vi "Init.vi"(8 "error in (no error)":errorcluster, 11 "Laser View in":refnum<class "Laser View.lvclass">) -> (0 "error out":errorcluster, 3 "Laser View out":refnum<class "Laser View.lvclass">)   [LabVIEW 2022 SP3, in "Laser View.lvclass"]
uses:
  Laser View.lvclass
  Data.ctl
  Laser View.lvclass/Laser View.ctl
  iView/base view/base view.lvclass
  Laser Controller api/Laser API.lvclass
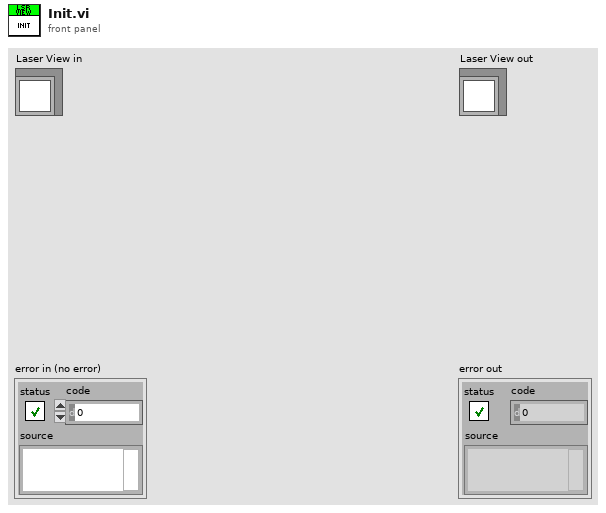
[diagram p1: front panel]
types:
  T1 = typedef "Laser View.lvclass/Data.ctl" = cluster{"Laser API.lvclass":refnum<class "Laser API.lvclass">}
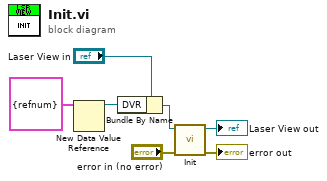
[diagram p0: block diagram]
diagram:
  n1 = New Data Value Reference(data value=T1 {"Laser API.lvclass"=refnum} ("Data")) -> (data value reference=w1:refnum<data-value>)  [unwired: 1 in, 1 out]
  n2 = Bundle By Name(cluster="Laser View in", "DVR"=w1) -> (w2:refnum<class "Laser View.lvclass">)
  n3 = call-parent "Init.vi"("error in (no error)"="error in (no error)", "base view in"=w2) -> ("error out"=→"error out":errorcluster, "base view out"=→"Laser View out":refnum<class "Laser View.lvclass">)  [unwired: 8 in]
